vi "BASE-Main.vi"() -> ()   [LabVIEW 2017]
uses:
  55ed0eea-cd20-493f-8468-85b8c1a0a0c0.vi
  <vilib>/Utility/error.llb/DialogType.ctl
panel:
  in  "Table Drawing":bool
  in  "Setting":bool
  in  "Manual":bool
  in  "I/O SCREEN":bool
  out "Status Number":i32
  out "Status":i32(ring)=1 items=["Stopped"=1, "StartPending"=2, "StopPending"=3, "Running"=4, "ContinuePending"=5, "PausePending"=6, "Paused"=7]
  in  "RECIPE":bool
  out "error out":errorcluster
  in  "Logout":bool
  in  "Stop":bool
  in  "Create Login":bool
  in  "Reports":bool
  in  "Start":bool
  out "Time":string
  out "Date":string
  in  "Login":bool
  # "CKD"
types:
  T1 = enum8{"Enabled", "Disabled", "Disabled and Grayed Out"}
  T2 = enum32{"Invalid", "Standard", "Closed", "Hidden", "Minimized", "Maximized"}
  T3 = typedef "DialogType.ctl" = u16
  T4 = enum32{"invalid app kind", "Development System", "Run Time System", "Student Edition", "Embedded LabVIEW", "Evaluation", "Custom"}
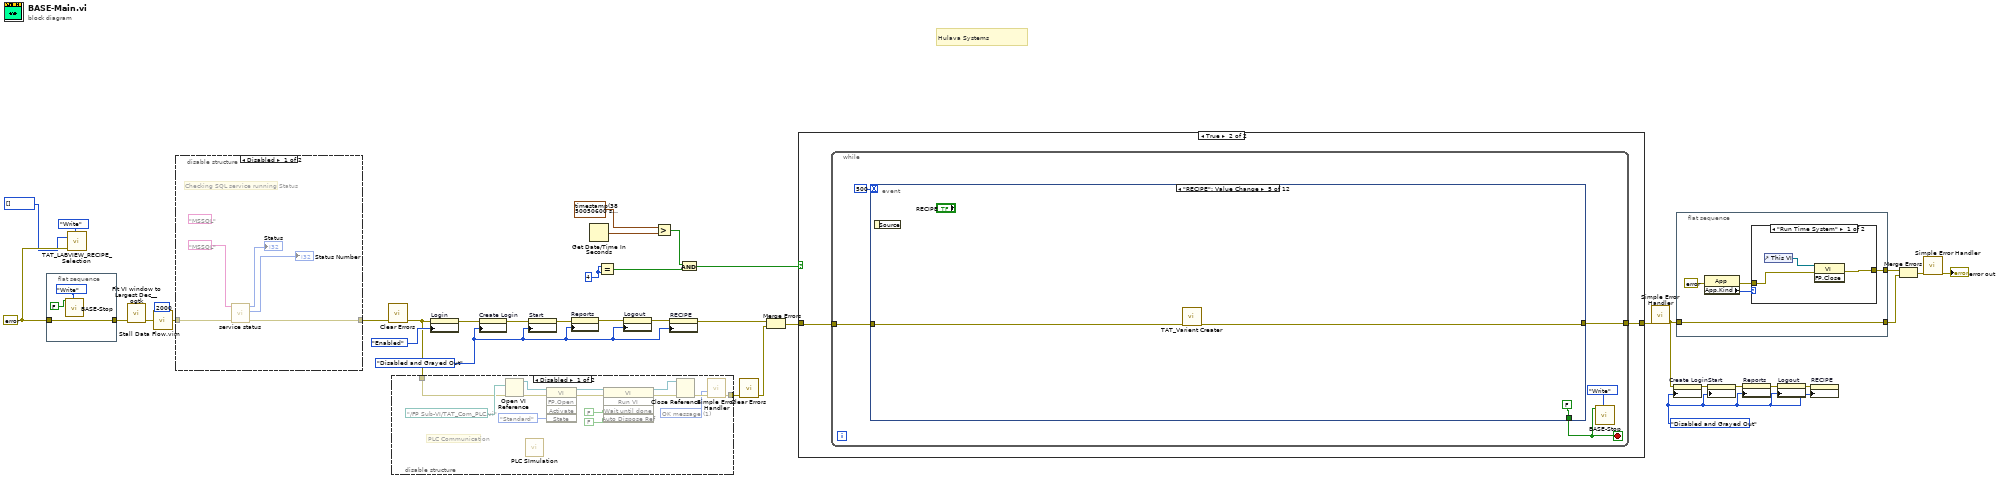
[diagram p0: block diagram]
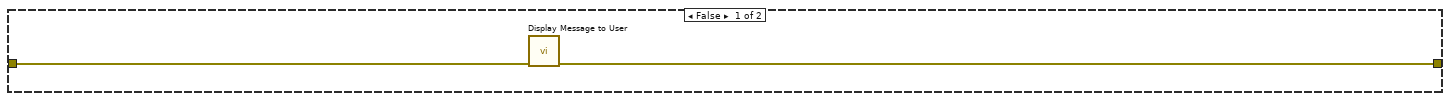
[diagram p5: hidden frame]
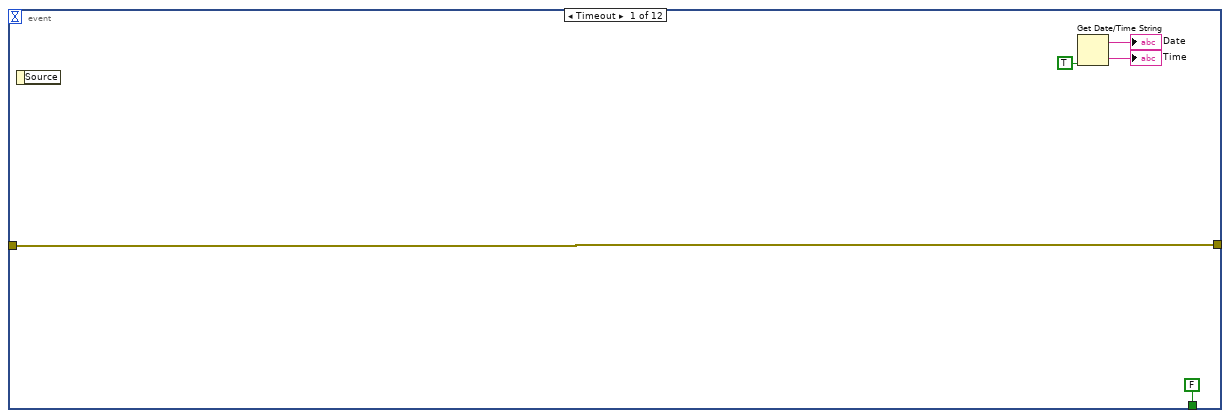
[diagram p6: hidden frame]
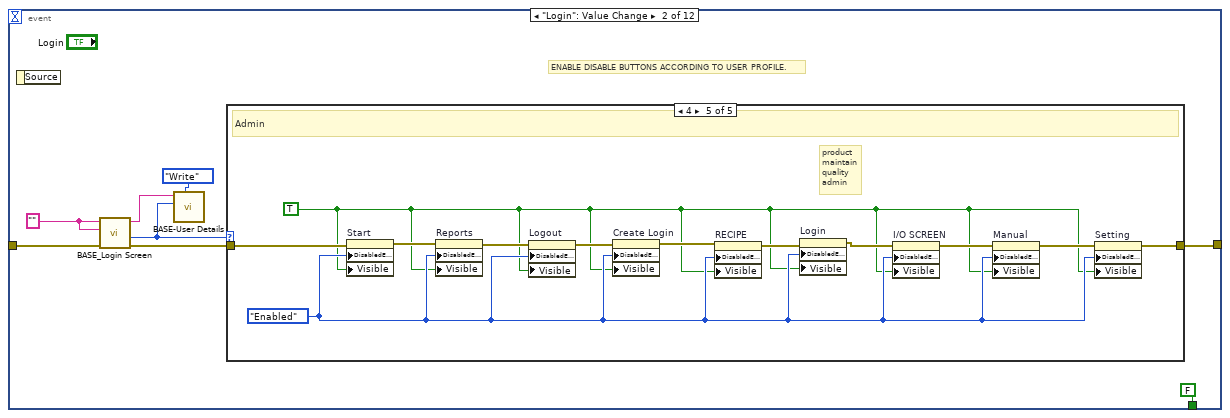
[diagram p7: hidden frame]
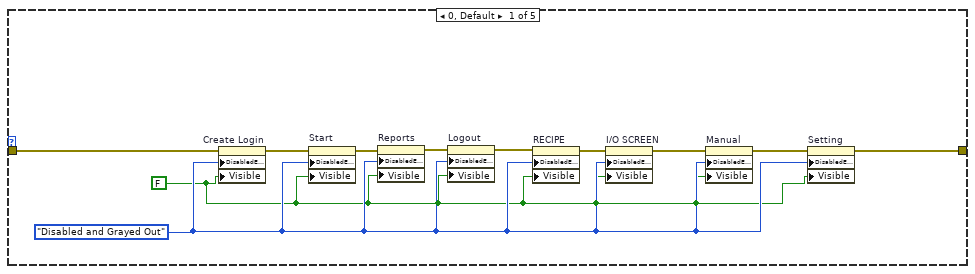
[diagram p8: hidden frame]
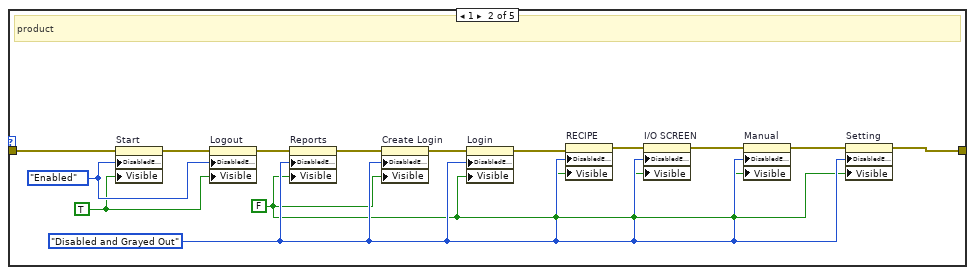
[diagram p9: hidden frame]
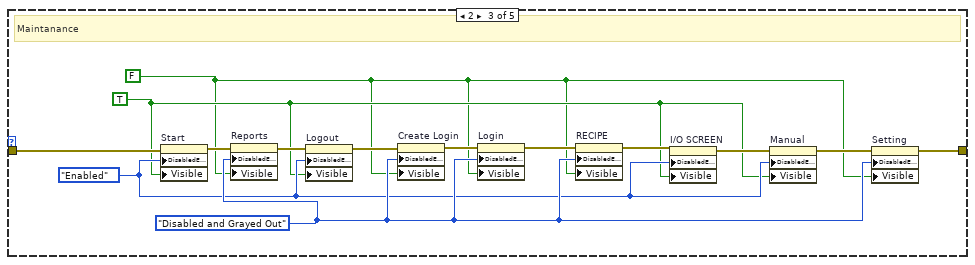
[diagram p10: hidden frame]
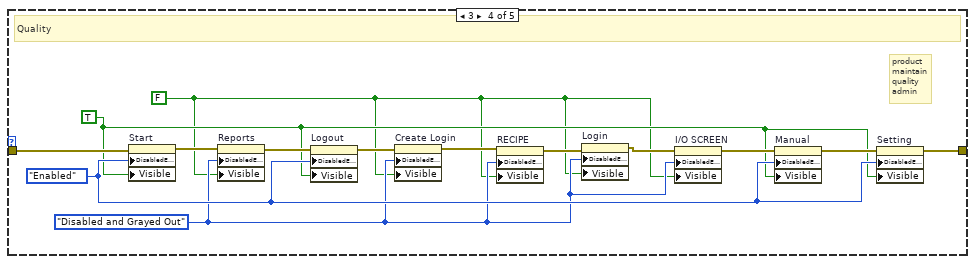
[diagram p11: hidden frame]
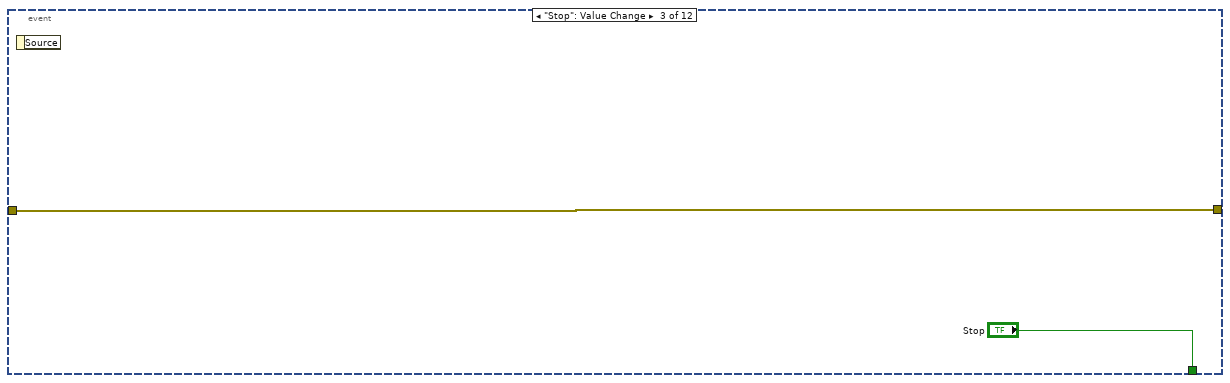
[diagram p12: hidden frame]
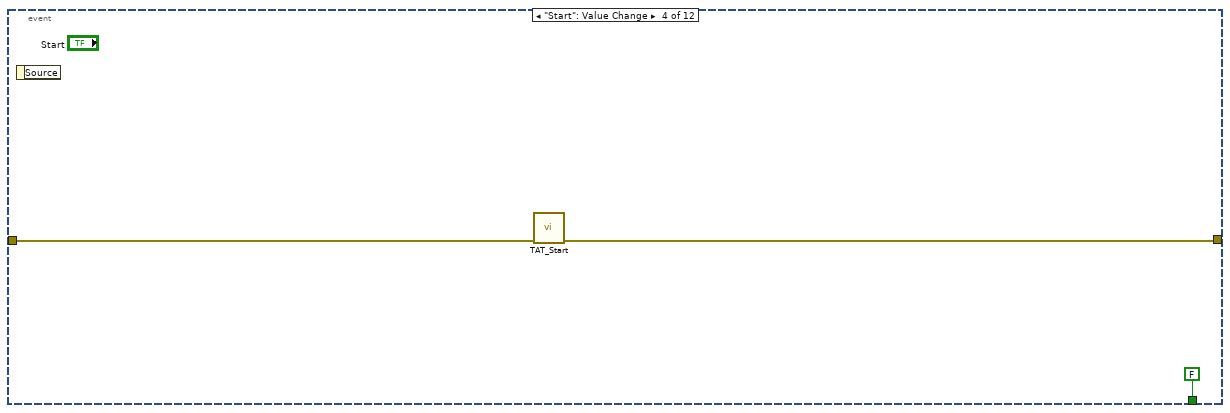
[diagram p13: hidden frame]
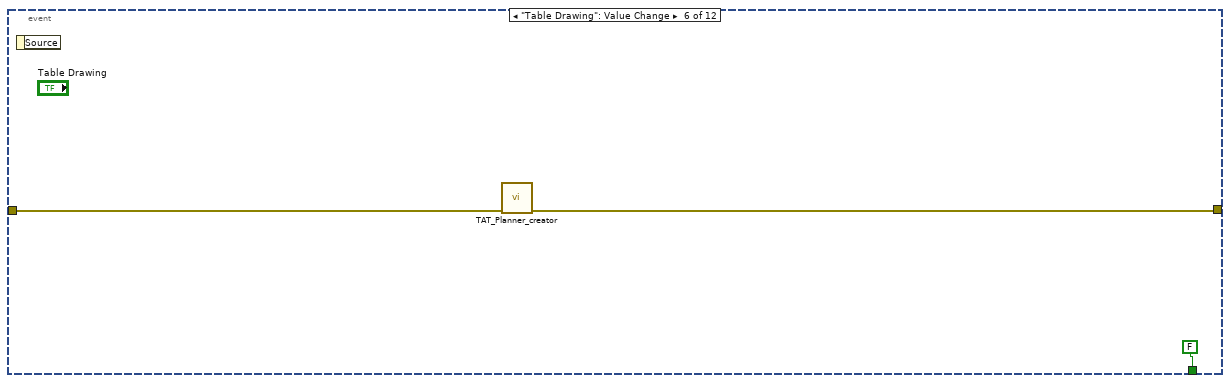
[diagram p14: hidden frame]
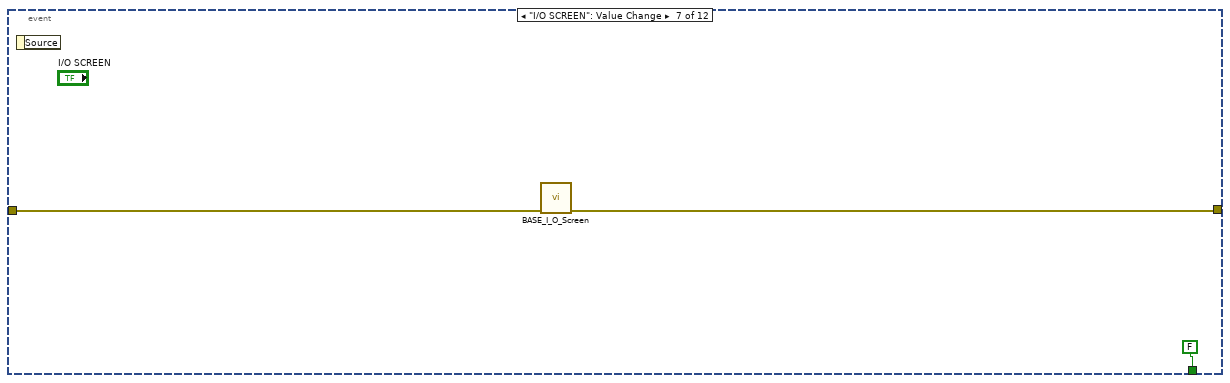
[diagram p15: hidden frame]
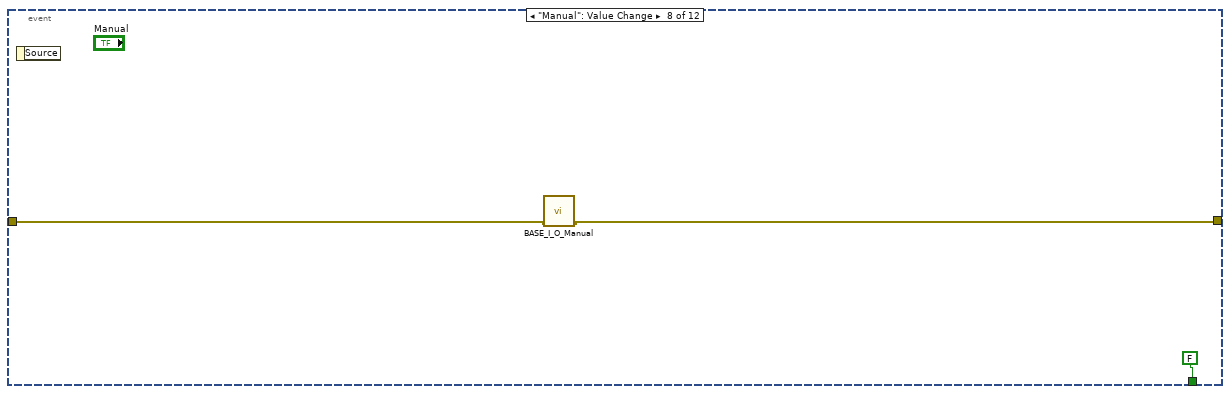
[diagram p16: hidden frame]
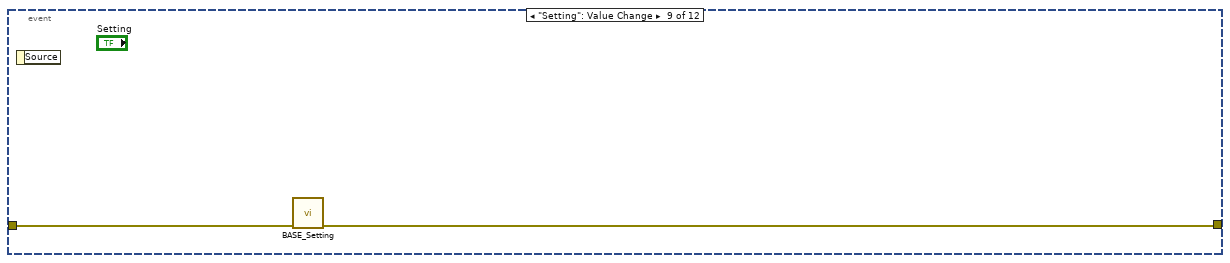
[diagram p17: hidden frame]
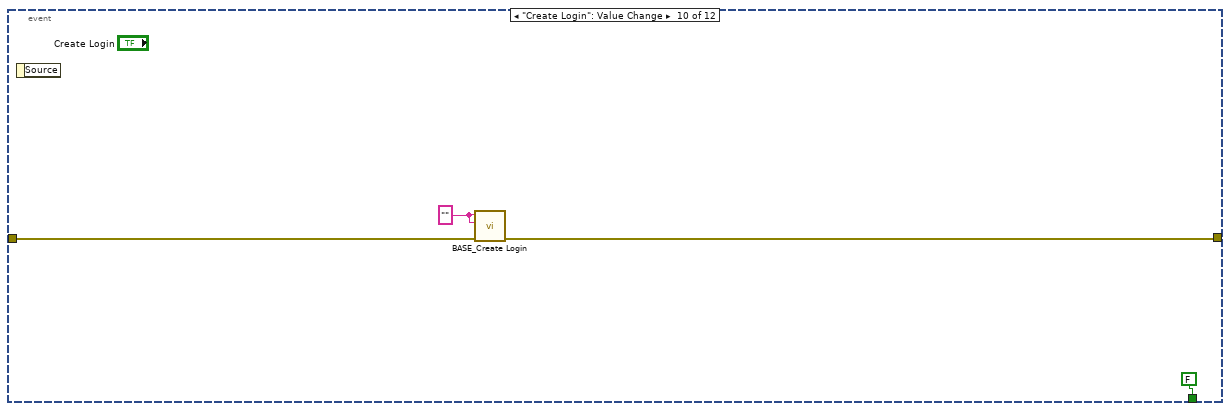
[diagram p18: hidden frame]
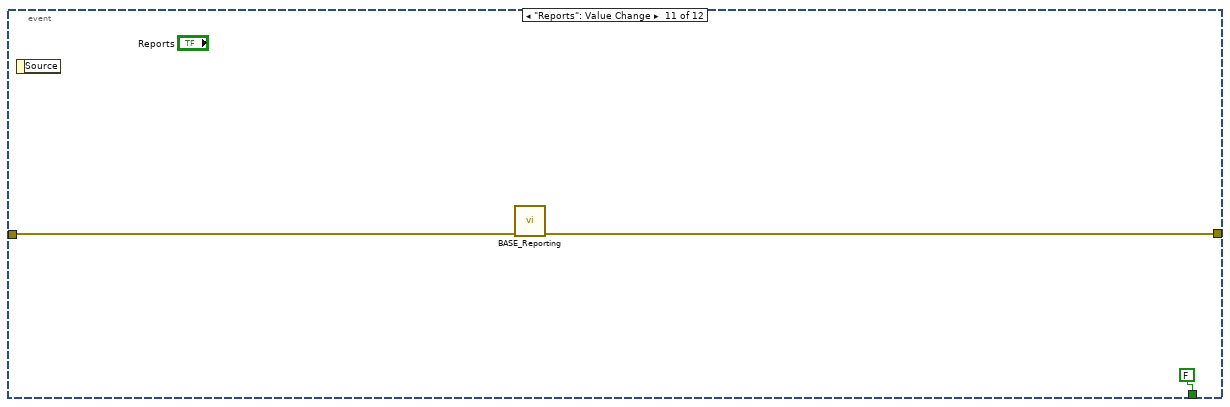
[diagram p19: hidden frame]
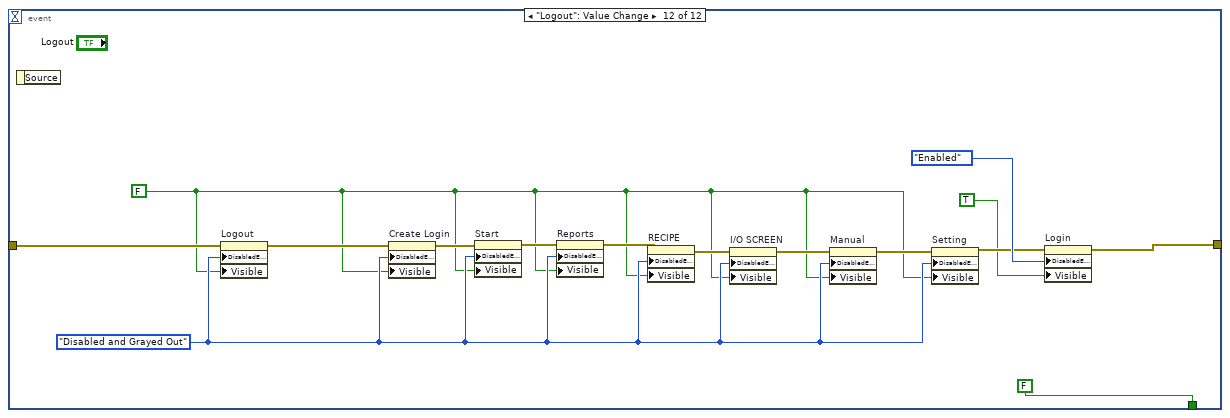
[diagram p20: hidden frame]
diagram:
  w11 = T1."Disabled and Grayed Out" ("Disabled")
  w2 = 4 ("y")
  w3 = errorcluster {"status"=FALSE, "code"=0, "source"=""} ("error constant")
  w12 = T1."Disabled and Grayed Out" ("Disabled")
  # "Hulava Systems"
  n1 = flat-sequence {
    tunnel: [w40] -> w28
    tunnel: w3 -> [w40]
    frame #0 {
      n2 = call "BASE-Stop.vi"("Enum"=enum16{"Read", "Write"}."Write", "Stop"=FALSE) -> ()  [unwired: 9 in, 1 out]
    }
  }
  n3 = call "TAT_LABVIEW_RECIPE_Selection.vi"("Enum"=enum16{"Read", "Write"}."Write", "error in (no error)"=w3, "in"=i32[] []) -> ()  [unwired: 7 in, 2 out]
  n4 = call <userlib>:"Fit VI window to Largest Dec__ogtk.vi"("error in (no error)"=w28) -> ("error out"=w17:errorcluster)  [unwired: 5 in, 1 out]
  n5 = call "Stall Data Flow.vim"("value in"=w17, "milliseconds to wait"=u32 2000) -> ("value out"=w16:errorcluster)  [unwired: 1 out]
  n6 = disable-structure shown="Disabled" {
    disable-tunnel: [w42 w46] -> w24
    disable-tunnel: w16 -> [w41 w46]
    frame Disabled {
      (unwired) "MSSQL" ("Service Name")
      # "Checking SQL service running Status"
      n7 = call "service status.vi"("error in"=w41, "Service Name"="MSSQL") -> ("error out"=w42:errorcluster, "Status Number"=→"Status Number":i32, "Status"=→"Status":i32)  [unwired: 6 in, 1 out]
    }
    frame Enabled {
    }
  }
  n8 = call <vilib>:"Clear Errors.vi"("error in (no error)"=w24) -> ("error out"=w23:errorcluster)  [unwired: 5 in, 1 out]
  n9 = disable-structure shown="Disabled" {
    disable-tunnel: [w48 w61] -> w26
    disable-tunnel: w23 -> [w47 w61]
    frame Disabled {
      w49 = T3 1 items=["no dialog", "OK message", "continue or stop message", "OK message + warnings", "continue/stop + warnings"] ("type of dialog (OK msg:1)")
      # "PLC Communication"
      n10 = Open VI Reference(vi path=path "../FP Sub-VI/TAT_Com_PLC.vi", error in (no error)=w47) -> (vi reference=w57:refnum<vi>, error out=w58:errorcluster)  [unwired: 4 in]
      n11 = call "PLC SImulation.vi"() -> ()  [unwired: 12 in]
      n12 = invoke class="VI" method="FP.Open"(reference=w57, error in=w58, "State"=T2."Standard") -> (reference out=w60:refnum<vi>, error out=w59:errorcluster)  [unwired: 2 in, 3 out]
      n13 = invoke class="VI" method="Run VI"(reference=w60, error in=w59, "Wait until done"=FALSE ("Wait Until Done"), "Auto Dispose Ref"=FALSE ("Auto Dispose Reference")) -> (reference out=w56:refnum<vi>, error out=w55:errorcluster)  [unwired: 1 in, 3 out]
      n14 = Close Reference(reference=w56, error in (no error)=w55) -> (error out=w50:errorcluster)
      n15 = call <vilib>:"Simple Error Handler.vi"("type of dialog (OK msg:1)"=w49, "error in (no error)"=w50) -> ("error out"=w48:errorcluster)  [unwired: 3 in, 4 out]
    }
    frame Enabled {
    }
  }
  n16 = property on="Login" class="Bool"(error in=w23, "DisabledEnum"=T1."Enabled" ("Disabled")) -> (error out=w32:errorcluster)  [unwired: 1 in, 1 out]
  n17 = property on="Create Login" class="Bool"(error in=w32, "DisabledEnum"=w12) -> (error out=w36:errorcluster)  [unwired: 1 in, 1 out]
  n18 = property on="Start" class="Bool"(error in=w36, "DisabledEnum"=w12) -> (error out=w13:errorcluster)  [unwired: 1 in, 1 out]
  n19 = property on="Reports" class="Bool"(error in=w13, "DisabledEnum"=w12) -> (error out=w30:errorcluster)  [unwired: 1 in, 1 out]
  n20 = Get Date/Time In Seconds() -> (seconds since 1Jan1904=w19:timestamp)
  n21 = Equal?(x=w2, y=w2) -> (x = y?=w22:bool)
  n22 = property on="Logout" class="Bool"(error in=w30, "DisabledEnum"=w12) -> (error out=w14:errorcluster)  [unwired: 1 in, 1 out]
  n23 = Greater?(x=timestamp(3850050600 s since 1904-01-01), y=w19) -> (0:w18:bool)
  n24 = property on="RECIPE" class="Bool"(error in=w14, "DisabledEnum"=w12) -> (error out=w5:errorcluster)  [unwired: 1 in, 1 out]
  n25 = And(x=w18, y=w22) -> (x .and. y?=w21:bool)
  n26 = call <vilib>:"Clear Errors.vi"("error in (no error)"=w26) -> ("error out"=w25:errorcluster)  [unwired: 5 in, 1 out]
  n27 = Merge Errors(w5, w25) -> (w27:errorcluster)
  n28 = case shown="True" w21 {
    tunnel: w27 -> [w63 w65]
    tunnel: [w62 w64] -> w37
    frame False {
      n29 = call "Display Message to User"("error in (no error)"=w63) -> ("error out"=w62:errorcluster)  [unwired: 9 in, 1 out]
    }
    frame True {
      n30 = while {
        tunnel: w65 -> [w69]
        tunnel: [w68] -> w64
        stop <- w66 stop-if-true
        n31 = event shown="[4] \"RECIPE\": Value Change" {
          selector: _ -> [_ _ _ _ _ _ _ _ _ _ _ _]
          dyn-events: _ -> [_ _ _ _ _ _ _ _ _ _ _ _]
          timeout: 500 -> [_ _ _ _ _ _ _ _ _ _ _ _]
          tunnel: w69 -> [w73 w83 w149 w152 w155 w158 w161 w163 w167 w171 w173 w186]
          tunnel: [w73 w76 w149 w151 w154 w157 w160 w164 w166 w170 w172 w187] -> w68
          tunnel: [FALSE ("Stop") FALSE ("Stop") "Stop" FALSE ("Stop") FALSE ("Stop") FALSE ("Stop") FALSE ("Stop") FALSE ("Stop") _ FALSE ("Stop") FALSE ("Stop") FALSE ("Stop")] -> w66
          event Timeout {
            n32 = event-data() -> ()  [unwired: 1 in, 1 out]
            n33 = Get Date/Time String(want seconds? (F)=TRUE) -> (date string=→"Date":string, time string=→"Time":string)  [unwired: 2 in]
          }
          event "Login": Value Change {
            w79 = "" ("User Name")
            # "ENABLE DISABLE BUTTONS ACCORDING TO USER PROFILE."
            n34 = event-data() -> ()  [unwired: 1 in, 1 out]
            n35 = call "BASE_Login Screen.vi"("Error In"=w83, "Password"=w79, "User Name"=w79) -> ("error out"=w82:errorcluster, "Level"=w77:i32, "User Name Out"=w80:string)  [unwired: 5 in, 1 out]
            n36 = call "BASE-User Details.vi"("Enum"=enum16{"Read", "Write"}."Write", "Level In"=w77, "User Name In"=w80) -> ()  [unwired: 7 in, 2 out]
            n37 = case shown="4" w77 {
              tunnel: w82 -> [w92 w108 w122 w136 w148]
              tunnel: [w86 w100 w113 w128 w140] -> w76
              frame 0, Default {
                w84 = FALSE
                w85 = T1."Disabled and Grayed Out" ("Disabled")
                n38 = property on="Create Login" class="Bool"(error in=w92, "DisabledEnum"=w85, "Visible"=w84) -> (error out=w94:errorcluster)  [unwired: 1 in, 1 out]
                n39 = property on="Start" class="Bool"(error in=w94, "DisabledEnum"=w85, "Visible"=w84) -> (error out=w93:errorcluster)  [unwired: 1 in, 1 out]
                n40 = property on="Reports" class="Bool"(error in=w93, "DisabledEnum"=w85, "Visible"=w84) -> (error out=w90:errorcluster)  [unwired: 1 in, 1 out]
                n41 = property on="Logout" class="Bool"(error in=w90, "DisabledEnum"=w85, "Visible"=w84) -> (error out=w91:errorcluster)  [unwired: 1 in, 1 out]
                n42 = property on="RECIPE" class="Bool"(error in=w91, "DisabledEnum"=w85, "Visible"=w84) -> (error out=w87:errorcluster)  [unwired: 1 in, 1 out]
                n43 = property on="I/O SCREEN" class="Bool"(error in=w87, "DisabledEnum"=w85, "Visible"=w84) -> (error out=w89:errorcluster)  [unwired: 1 in, 1 out]
                n44 = property on="Manual" class="Bool"(error in=w89, "DisabledEnum"=w85, "Visible"=w84) -> (error out=w88:errorcluster)  [unwired: 1 in, 1 out]
                n45 = property on="Setting" class="Bool"(error in=w88, "DisabledEnum"=w85, "Visible"=w84) -> (error out=w86:errorcluster)  [unwired: 1 in, 1 out]
              }
              frame 1 {
                w95 = FALSE
                w96 = TRUE
                w97 = T1."Disabled and Grayed Out" ("Disabled")
                w102 = T1."Enabled" ("Disabled")
                # "product"
                n46 = property on="Start" class="Bool"(error in=w108, "DisabledEnum"=w102, "Visible"=w96) -> (error out=w104:errorcluster)  [unwired: 1 in, 1 out]
                n47 = property on="Logout" class="Bool"(error in=w104, "DisabledEnum"=w102, "Visible"=w96) -> (error out=w106:errorcluster)  [unwired: 1 in, 1 out]
                n48 = property on="Reports" class="Bool"(error in=w106, "DisabledEnum"=w97, "Visible"=w95) -> (error out=w107:errorcluster)  [unwired: 1 in, 1 out]
                n49 = property on="Create Login" class="Bool"(error in=w107, "DisabledEnum"=w97, "Visible"=w95) -> (error out=w105:errorcluster)  [unwired: 1 in, 1 out]
                n50 = property on="Login" class="Bool"(error in=w105, "DisabledEnum"=w97, "Visible"=w95) -> (error out=w103:errorcluster)  [unwired: 1 in, 1 out]
                n51 = property on="RECIPE" class="Bool"(error in=w103, "DisabledEnum"=w97, "Visible"=w95) -> (error out=w98:errorcluster)  [unwired: 1 in, 1 out]
                n52 = property on="I/O SCREEN" class="Bool"(error in=w98, "DisabledEnum"=w97, "Visible"=w95) -> (error out=w99:errorcluster)  [unwired: 1 in, 1 out]
                n53 = property on="Manual" class="Bool"(error in=w99, "DisabledEnum"=w97, "Visible"=w95) -> (error out=w101:errorcluster)  [unwired: 1 in, 1 out]
                n54 = property on="Setting" class="Bool"(error in=w101, "DisabledEnum"=w97, "Visible"=w95) -> (error out=w100:errorcluster)  [unwired: 1 in, 1 out]
              }
              frame 2 {
                w109 = FALSE
                w110 = TRUE
                w112 = T1."Disabled and Grayed Out" ("Disabled")
                w111 = T1."Enabled" ("Disabled")
                # "Maintanance"
                n55 = property on="Start" class="Bool"(error in=w122, "DisabledEnum"=w111, "Visible"=w110) -> (error out=w119:errorcluster)  [unwired: 1 in, 1 out]
                n56 = property on="Reports" class="Bool"(error in=w119, "DisabledEnum"=w112, "Visible"=w109) -> (error out=w121:errorcluster)  [unwired: 1 in, 1 out]
                n57 = property on="Logout" class="Bool"(error in=w121, "DisabledEnum"=w111, "Visible"=w110) -> (error out=w117:errorcluster)  [unwired: 1 in, 1 out]
                n58 = property on="Create Login" class="Bool"(error in=w117, "DisabledEnum"=w112, "Visible"=w109) -> (error out=w120:errorcluster)  [unwired: 1 in, 1 out]
                n59 = property on="Login" class="Bool"(error in=w120, "DisabledEnum"=w112, "Visible"=w109) -> (error out=w118:errorcluster)  [unwired: 1 in, 1 out]
                n60 = property on="RECIPE" class="Bool"(error in=w118, "DisabledEnum"=w112, "Visible"=w109) -> (error out=w114:errorcluster)  [unwired: 1 in, 1 out]
                n61 = property on="I/O SCREEN" class="Bool"(error in=w114, "DisabledEnum"=w111, "Visible"=w110) -> (error out=w115:errorcluster)  [unwired: 1 in, 1 out]
                n62 = property on="Manual" class="Bool"(error in=w115, "DisabledEnum"=w111, "Visible"=w110) -> (error out=w116:errorcluster)  [unwired: 1 in, 1 out]
                n63 = property on="Setting" class="Bool"(error in=w116, "DisabledEnum"=w112, "Visible"=w109) -> (error out=w113:errorcluster)  [unwired: 1 in, 1 out]
              }
              frame 3 {
                w123 = FALSE
                w124 = TRUE
                w125 = T1."Disabled and Grayed Out" ("Disabled")
                w126 = T1."Enabled" ("Disabled")
                # "product\nmaintain\nquality\nadmin"
                # "Quality"
                n64 = property on="Start" class="Bool"(error in=w136, "DisabledEnum"=w126, "Visible"=w124) -> (error out=w131:errorcluster)  [unwired: 1 in, 1 out]
                n65 = property on="Reports" class="Bool"(error in=w131, "DisabledEnum"=w125, "Visible"=w123) -> (error out=w135:errorcluster)  [unwired: 1 in, 1 out]
                n66 = property on="Logout" class="Bool"(error in=w135, "DisabledEnum"=w126, "Visible"=w124) -> (error out=w134:errorcluster)  [unwired: 1 in, 1 out]
                n67 = property on="Create Login" class="Bool"(error in=w134, "DisabledEnum"=w125, "Visible"=w123) -> (error out=w133:errorcluster)  [unwired: 1 in, 1 out]
                n68 = property on="RECIPE" class="Bool"(error in=w133, "DisabledEnum"=w125, "Visible"=w123) -> (error out=w132:errorcluster)  [unwired: 1 in, 1 out]
                n69 = property on="Login" class="Bool"(error in=w132, "DisabledEnum"=w125, "Visible"=w123) -> (error out=w127:errorcluster)  [unwired: 1 in, 1 out]
                n70 = property on="I/O SCREEN" class="Bool"(error in=w127, "DisabledEnum"=w125, "Visible"=w123) -> (error out=w129:errorcluster)  [unwired: 1 in, 1 out]
                n71 = property on="Manual" class="Bool"(error in=w129, "DisabledEnum"=w126, "Visible"=w124) -> (error out=w130:errorcluster)  [unwired: 1 in, 1 out]
                n72 = property on="Setting" class="Bool"(error in=w130, "DisabledEnum"=w126, "Visible"=w124) -> (error out=w128:errorcluster)  [unwired: 1 in, 1 out]
              }
              frame 4 {
                w137 = TRUE
                w138 = T1."Enabled" ("Disabled")
                # "product\nmaintain\nquality\nadmin"
                # "Admin"
                n73 = property on="Start" class="Bool"(error in=w148, "DisabledEnum"=w138, "Visible"=w137) -> (error out=w143:errorcluster)  [unwired: 1 in, 1 out]
                n74 = property on="Reports" class="Bool"(error in=w143, "DisabledEnum"=w138, "Visible"=w137) -> (error out=w147:errorcluster)  [unwired: 1 in, 1 out]
                n75 = property on="Logout" class="Bool"(error in=w147, "DisabledEnum"=w138, "Visible"=w137) -> (error out=w146:errorcluster)  [unwired: 1 in, 1 out]
                n76 = property on="Create Login" class="Bool"(error in=w146, "DisabledEnum"=w138, "Visible"=w137) -> (error out=w145:errorcluster)  [unwired: 1 in, 1 out]
                n77 = property on="RECIPE" class="Bool"(error in=w145, "DisabledEnum"=w138, "Visible"=w137) -> (error out=w144:errorcluster)  [unwired: 1 in, 1 out]
                n78 = property on="Login" class="Bool"(error in=w144, "DisabledEnum"=w138, "Visible"=w137) -> (error out=w139:errorcluster)  [unwired: 1 in, 1 out]
                n79 = property on="I/O SCREEN" class="Bool"(error in=w139, "DisabledEnum"=w138, "Visible"=w137) -> (error out=w141:errorcluster)  [unwired: 1 in, 1 out]
                n80 = property on="Manual" class="Bool"(error in=w141, "DisabledEnum"=w138, "Visible"=w137) -> (error out=w142:errorcluster)  [unwired: 1 in, 1 out]
                n81 = property on="Setting" class="Bool"(error in=w142, "DisabledEnum"=w138, "Visible"=w137) -> (error out=w140:errorcluster)  [unwired: 1 in, 1 out]
              }
            }
          }
          event "Stop": Value Change {
            n82 = event-data() -> ()  [unwired: 1 in, 1 out]
          }
          event "Start": Value Change {
            n83 = event-data() -> ()  [unwired: 1 in, 1 out]
            n84 = call "TAT_Start.vi"("error In"=w152) -> ("error out"=w151:errorcluster)  [unwired: 10 in]
          }
          event "RECIPE": Value Change {
            n85 = event-data() -> ()  [unwired: 1 in, 1 out]
            n86 = call "TAT_Varient Creater.vi"("error in (no error)"=w155) -> ("error out"=w154:errorcluster)  [unwired: 10 in]
          }
          event "Table Drawing": Value Change {
            n87 = event-data() -> ()  [unwired: 1 in, 1 out]
            n88 = call "TAT_Planner_creator.vi"("error in (no error)"=w158) -> ("error out"=w157:errorcluster)  [unwired: 10 in]
          }
          event "I/O SCREEN": Value Change {
            n89 = event-data() -> ()  [unwired: 1 in, 1 out]
            n90 = call "BASE_I_O_Screen.vi"("error in (no error)"=w161) -> ("error out"=w160:errorcluster)  [unwired: 10 in]
          }
          event "Manual": Value Change {
            n91 = event-data() -> ()  [unwired: 1 in, 1 out]
            n92 = call "BASE_I_O_Manual.vi"("error in (no error)"=w163) -> ("error out"=w164:errorcluster)  [unwired: 10 in]
          }
          event "Setting": Value Change {
            n93 = event-data() -> ()  [unwired: 1 in, 1 out]
            n94 = call "BASE_Setting.vi"("error in (no error)"=w167) -> ("error out"=w166:errorcluster)  [unwired: 10 in]
          }
          event "Create Login": Value Change {
            w169 = "" ("User Name")
            n95 = event-data() -> ()  [unwired: 1 in, 1 out]
            n96 = call "BASE_Create Login.vi"("Error In"=w171, "Password"=w169, "User Name"=w169) -> ("error out"=w170:errorcluster)  [unwired: 6 in]
          }
          event "Reports": Value Change {
            n97 = event-data() -> ()  [unwired: 1 in, 1 out]
            n98 = call "BASE_Reporting.vi"("error in (no error)"=w173) -> ("error out"=w172:errorcluster)  [unwired: 10 in]
          }
          event "Logout": Value Change {
            w176 = FALSE
            w177 = T1."Disabled and Grayed Out" ("Disabled")
            n99 = event-data() -> ()  [unwired: 1 in, 1 out]
            n100 = property on="Logout" class="Bool"(error in=w186, "DisabledEnum"=w177, "Visible"=w176) -> (error out=w182:errorcluster)  [unwired: 1 in, 1 out]
            n101 = property on="Create Login" class="Bool"(error in=w182, "DisabledEnum"=w177, "Visible"=w176) -> (error out=w189:errorcluster)  [unwired: 1 in, 1 out]
            n102 = property on="Start" class="Bool"(error in=w189, "DisabledEnum"=w177, "Visible"=w176) -> (error out=w188:errorcluster)  [unwired: 1 in, 1 out]
            n103 = property on="Reports" class="Bool"(error in=w188, "DisabledEnum"=w177, "Visible"=w176) -> (error out=w183:errorcluster)  [unwired: 1 in, 1 out]
            n104 = property on="RECIPE" class="Bool"(error in=w183, "DisabledEnum"=w177, "Visible"=w176) -> (error out=w178:errorcluster)  [unwired: 1 in, 1 out]
            n105 = property on="I/O SCREEN" class="Bool"(error in=w178, "DisabledEnum"=w177, "Visible"=w176) -> (error out=w180:errorcluster)  [unwired: 1 in, 1 out]
            n106 = property on="Manual" class="Bool"(error in=w180, "DisabledEnum"=w177, "Visible"=w176) -> (error out=w181:errorcluster)  [unwired: 1 in, 1 out]
            n107 = property on="Setting" class="Bool"(error in=w181, "DisabledEnum"=w177, "Visible"=w176) -> (error out=w179:errorcluster)  [unwired: 1 in, 1 out]
            n108 = property on="Login" class="Bool"(error in=w179, "DisabledEnum"=T1."Enabled" ("Disabled"), "Visible"=TRUE) -> (error out=w187:errorcluster)  [unwired: 1 in, 1 out]
          }
        }
        n109 = call "BASE-Stop.vi"("Enum"=enum16{"Read", "Write"}."Write", "Stop"=w66) -> ()  [unwired: 9 in, 1 out]
      }
    }
  }
  n110 = call <vilib>:"Simple Error Handler.vi"("error in (no error)"=w37) -> ("error out"=w6:errorcluster)  [unwired: 4 in, 4 out]
  n111 = property on="Create Login" class="Bool"(error in=w6, "DisabledEnum"=w11) -> (error out=w7:errorcluster)  [unwired: 1 in, 1 out]
  n112 = flat-sequence {
    tunnel: [w191] -> w35
    tunnel: [w190] -> w33
    tunnel: w6 -> [w190]
    frame #0 {
      n113 = property class="App"(error in=errorcluster {"status"=FALSE, "code"=0, "source"=""} ("error in (no error)")) -> (error out=w193:errorcluster, "App.Kind"=w194:T4)  [unwired: 1 in, 1 out]
      n114 = case shown="\"Run Time System\"" w194 {
        tunnel: w193 -> [w196 w198]
        tunnel: [w195 w198] -> w191
        frame "Run Time System" {
          n115 = control-ref of="This VI"() -> (w197:refnum<vi>)
          n116 = invoke class="VI" method="FP.Close"(reference=w197, error in=w196) -> (error out=w195:errorcluster)  [unwired: 1 in, 2 out]
        }
        frame "Development System", Default {
        }
      }
    }
  }
  n117 = property on="Start" class="Bool"(error in=w7, "DisabledEnum"=w11) -> (error out=w10:errorcluster)  [unwired: 1 in, 1 out]
  n118 = property on="Reports" class="Bool"(error in=w10, "DisabledEnum"=w11) -> (error out=w8:errorcluster)  [unwired: 1 in, 1 out]
  n119 = property on="Logout" class="Bool"(error in=w8, "DisabledEnum"=w11) -> (error out=w9:errorcluster)  [unwired: 1 in, 1 out]
  n120 = property on="RECIPE" class="Bool"(error in=w9, "DisabledEnum"=w11) -> ()  [unwired: 1 in, 2 out]
  n121 = Merge Errors(w35, w33) -> (w34:errorcluster)
  n122 = call <vilib>:"Simple Error Handler.vi"("error in (no error)"=w34) -> ("error out"=→"error out":errorcluster)  [unwired: 4 in, 4 out]
